vi "Yaw Crossover.vi"(9 "Target Yaw":dbl, 10 "Yaw in":dbl, 11 "Adjustment":dbl) -> (3 "Numeric out":dbl)   [LabVIEW 2017]
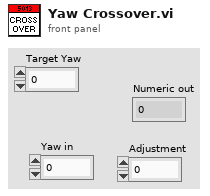
[diagram p1: front panel]
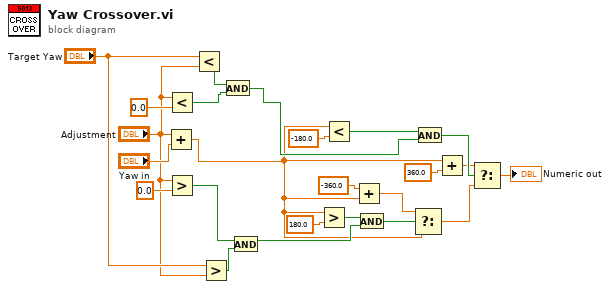
[diagram p0: block diagram]
diagram:
  n1 = Add(x="Adjustment", y="Yaw in") -> (x+y=w2:dbl)
  n2 = Less?(x="Adjustment", y=0.0 ("Y-Axis")) -> (x < y?=w8:bool)
  n3 = Greater?(x="Adjustment", y=0.0 ("Y-Axis")) -> (0:w9:bool)
  n4 = Less?(x="Target Yaw", y="Adjustment") -> (x < y?=w6:bool)
  n5 = Greater?(x="Target Yaw", y="Adjustment") -> (0:w4:bool)
  n6 = And(x=w6, y=w8) -> (x .and. y?=w7:bool)
  n7 = And(x=w9, y=w4) -> (x .and. y?=w5:bool)
  n8 = Greater?(x=w2, y=180.0) -> (0:w18:bool)
  n9 = Less?(x=w2, y=-180.0) -> (x < y?=w23:bool)
  n10 = Add(x=-360.0, y=w2) -> (x+y=w15:dbl)
  n11 = And(x=w18, y=w5) -> (x .and. y?=w17:bool)
  n12 = Select(t=w15, s=w17, f=w2) -> (s? t:f=w14:dbl)
  n13 = And(x=w23, y=w7) -> (x .and. y?=w22:bool)
  n14 = Add(x=w2, y=360.0) -> (x+y=w20:dbl)
  n15 = Select(t=w20, s=w22, f=w14) -> (s? t:f=→"Numeric out":dbl)
